vi "SetParam.vi"(8 "error in (no error)":errorcluster caption="entrée d'erreur (pas d'erreur)", 10 "MissingIndicator":T1={"missing_values"="nan", "features"="None", "sparse"="None", "error_on_new"=TRUE}, 11 "MissingIndicator.lvclass":refnum<class "MissingIndicator.lvclass">) -> (0 "error out":errorcluster caption="sortie d'erreur", 3 "MissingIndicator.lvclass":refnum<class "MissingIndicator.lvclass">)   [LabVIEW 2020, in "MissingIndicator.lvclass"]
doc: "Set Parameters"
uses:
  MissingIndicator.lvclass
  MissingIndicator.lvclass/MissingIndicator.ctl
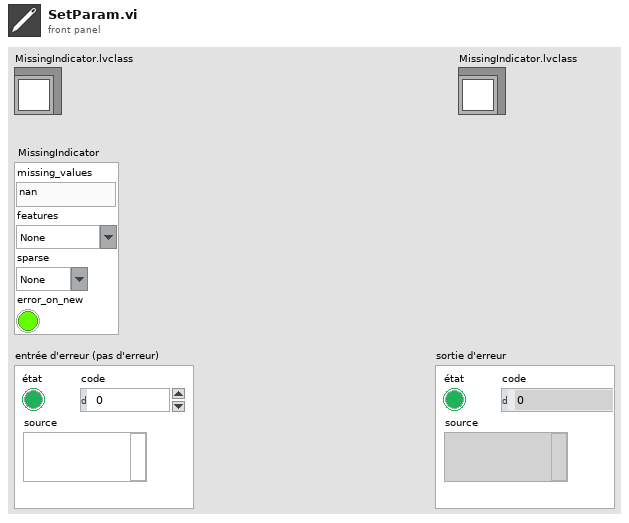
[diagram p1: front panel]
types:
  T1 = cluster{"missing_values":string, "features":string, "sparse":string, "error_on_new":bool}
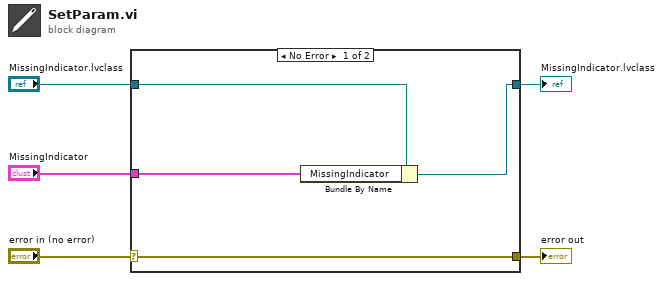
[diagram p0: block diagram]
diagram:
  n1 = case shown="No Error" "error in (no error)" {
    selector: "error in (no error)" -> [w9 w10]
    tunnel: [w9 w10] -> w4
    tunnel: [w7 w11] -> w2
    tunnel: "MissingIndicator.lvclass" -> [w8 w11]
    tunnel: "MissingIndicator" -> [w6 _]
    frame No Error {
      n2 = Bundle By Name(cluster=w8, "MissingIndicator"=w6) -> (w7:refnum<class "MissingIndicator.lvclass">)
    }
    frame Error {
    }
  }
  "error out" <- w4
  "MissingIndicator.lvclass" <- w2
